vi "Run.vi"(7 "Team Index":i32, 8 "Column":i32, 9 "Row":i32, 10 "View":i32[](array[numeric]) caption="View (Team Index, -1: empty)", 11 "Template In":refnum<class "Demo.lvclass">) -> (0 "Replicated":refnum<class "Square.lvclass">, 1 "Direction":T1, 2 "Action":T2, 3 "Square Out":refnum<class "Square.lvclass">)   [LabVIEW 2015, in "Demo.lvclass"]
uses:
  Demo.lvclass
  Square/Square.lvclass
  Type Defs/Action Enum.ctl
  Type Defs/Direction Enum.ctl
  Demo.lvclass/Demo.ctl
  SubVIs/Read-Only Globals.vi
  SubVIs/Read-Only Stats.vi
  SubVIs/Globals (private).vi
  Type Defs/SB Type Defs.lvlib
  Common/Common.lvlib
panel:
  # "NW\nN\nNE\nE\nSE\nS\nSW\nW"
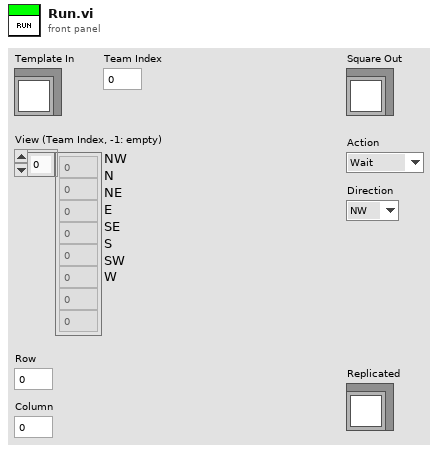
[diagram p1: front panel]
types:
  T1 = typedef "SB Type Defs.lvlib/Direction Enum.ctl" = enum16{"NW", "N", "NE", "E", "SE", "S", "SW", "W"}
  T2 = typedef "SB Type Defs.lvlib/Action Enum.ctl" = enum16{"Wait", "Move", "Attack", "Replicate"}
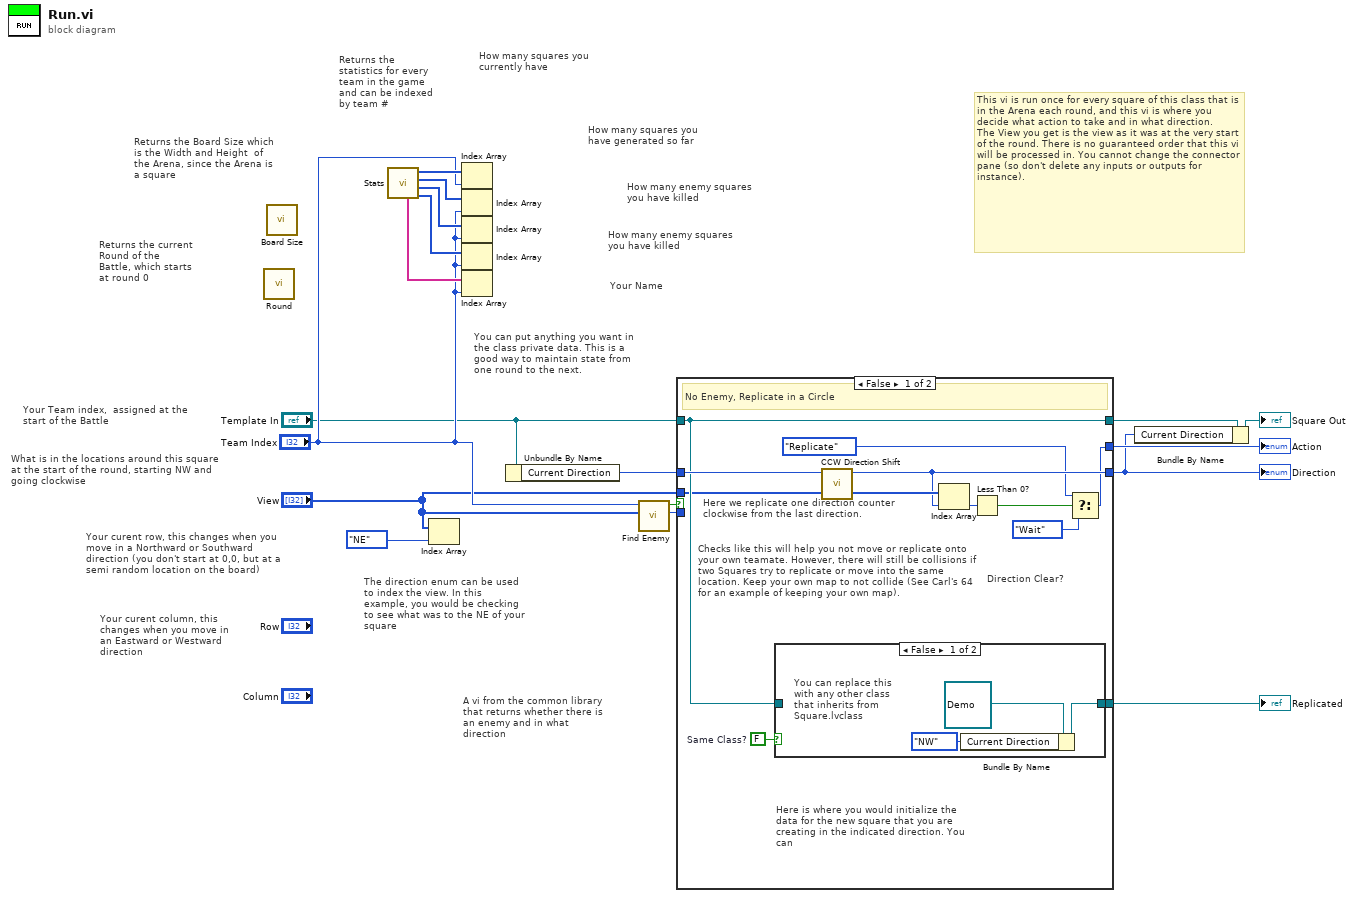
[diagram p0: block diagram]
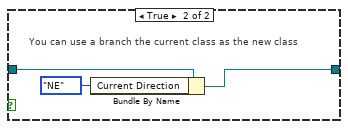
[diagram p2: hidden frame]
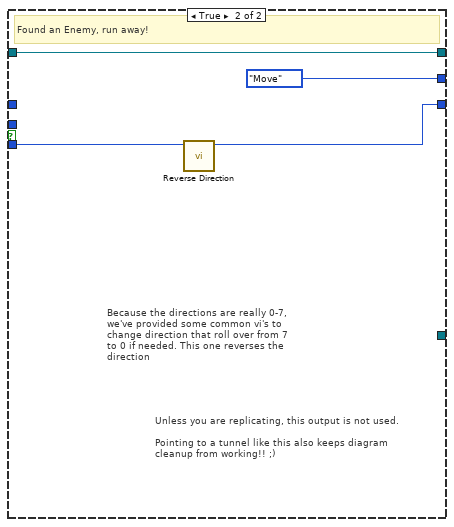
[diagram p3: hidden frame]
diagram:
  # "You can put anything you want in the class private data. This is a good way to maintain state from one round to the next."
  # "A vi from the common library that returns whether there is an enemy and in what direction"
  # "What is in the locations around this square at the start of the round, starting NW and going clockwise"
  # "Your Team index,  assigned at the start of the Battle"
  # "This vi is run once for every square of this class that is in the Arena each round, and this vi is where you decide what action to take and in what direction. \nThe View you get is the view as it was at the very start of the round. There is no guaranteed order that this vi will be processed in. You cannot change the connector pane (so don't delete any inputs or outputs for instance)."
  # "Your curent column, this changes when you move in an Eastward or Westward direction"
  # "Your curent row, this changes when you move in a Northward or Southward direction (you don't start at 0,0, but at a semi random location on the board)"
  # "The direction enum can be used to index the view. In this example, you would be checking to see what was to the NE of your square"
  # "Returns the Board Size which is the Width and Height  of the Arena, since the Arena is a square"
  # "Returns the current Round of the Battle, which starts at round 0"
  # "Returns the statistics for every team in the game  and can be indexed by team #"
  # "Your Name"
  # "How many enemy squares you have killed"
  # "How many enemy squares you have killed"
  # "How many squares you have generated so far"
  # "How many squares you currently have"
  n1 = call "Round.vi"() -> ()  [unwired: 11 in, 1 out]
  n2 = call "Board Size.vi"() -> ()  [unwired: 11 in, 1 out]
  n3 = call "Stats.vi"() -> ("Collisions"=w14:i32[], "Kills"=w15:i32[], "Generated"=w16:i32[], "Squares"=w17:i32[], "Players"=w13:string[])  [unwired: 7 in]
  n4 = Index Array(array="View", index=Direction_Enum."NE" ("Direction")) -> ()  [unwired: 1 out]
  n5 = Index Array(array=w17, index="Team Index") -> ()  [unwired: 1 out]
  n6 = Index Array(array=w16, index="Team Index") -> ()  [unwired: 1 out]
  n7 = Index Array(array=w15, index="Team Index") -> ()  [unwired: 1 out]
  n8 = Index Array(array=w14, index="Team Index") -> ()  [unwired: 1 out]
  n9 = Index Array(array=w13, index="Team Index") -> ()  [unwired: 1 out]
  n10 = Unbundle By Name("Template In") -> ("Current Direction"=w7:T1)
  n11 = call "Find Enemy.vi"("View"="View", "Team Index"="Team Index") -> ("Direction"=w9:T1, "Found Enemy?"=w10:bool)  [unwired: 7 in, 1 out]
  n12 = case shown="False" w10 {
    tunnel: w9 -> [_ w37]
    tunnel: [w19 Action_Enum."Move" ("Action")] -> w8
    tunnel: [w23 w36] -> w3
    tunnel: w7 -> [w28 _]
    tunnel: "Template In" -> [w27 w35]
    tunnel: [w27 w35] -> w5
    tunnel: [w26 _] -> w2
    tunnel: "View" -> [w24 _]
    frame False {
      w25 = FALSE  # Same Class?
      # "Direction Clear?"
      # "Checks like this will help you not move or replicate onto your own teamate. However, there will still be collisions if two Squares try to replicate or move into the same location. Keep your own map to not collide (See Carl's 64 for an example of keeping your own map)."
      # "Here is where you would initialize the data for the new square that you are creating in the indicated direction. You can"
      # "Here we replicate one direction counter clockwise from the last direction."
      # "No Enemy, Replicate in a Circle"
      n13 = case shown="False" w25 {
        tunnel: w27 -> [_ w34]
        tunnel: [w30 w33] -> w26
        frame False {
          # "You can replace this with any other class that inherits from Square.lvclass"
          n14 = Bundle By Name(cluster=refnum<class "Demo.lvclass"> refnum ("Template.lvclass"), "Current Direction"=Direction_Enum."NW") -> (w30:refnum<class "Demo.lvclass">)
        }
        frame True {
          # "You can use a branch the current class as the new class"
          n15 = Bundle By Name(cluster=w34, "Current Direction"=Direction_Enum."NE") -> (w33:refnum<class "Demo.lvclass">)
        }
      }
      n16 = call "CCW Direction Shift.vi"("Direction"=w28) -> ("Numeric"=w23:i32)  [unwired: 10 in]
      n17 = Index Array(array=w24, index=w23) -> (element=w22:i32)
      n18 = Less Than 0?(x=w22) -> (x < 0?=w21:bool)
      n19 = Select(t=Action_Enum."Replicate" ("Action"), s=w21, f=Action_Enum."Wait") -> (s? t:f=w19:T2)
    }
    frame True {
      # "Unless you are replicating, this output is not used. \n\nPointing to a tunnel like this also keeps diagram cleanup from working!! ;)"
      # "Because the directions are really 0-7, we've provided some common vi's to change direction that roll over from 7 to 0 if needed. This one reverses the direction"
      # "Found an Enemy, run away!"
      n20 = call "Reverse Direction.vi"("Direction in"=w37) -> ("Reverse Direction"=w36:i32)  [unwired: 10 in]
    }
  }
  "Action" <- w8
  "Direction" <- w3
  "Replicated" <- w2
  n21 = Bundle By Name(cluster=w5, "Current Direction"=w3) -> (→"Square Out":refnum<class "Demo.lvclass">)
